vi "4155C VAR2 StartStopStep to num steps.vi"(3 "step":dbl=0.01 format="%^.4e", 4 "stop":dbl=1.0 format="%^.4e", 5 "start":dbl format="%^.4e") -> (0 "Corrected Step":dbl format="%.2f", 1 "Number of points":i32=1, 2 "dup start":dbl format="%^.4e")   [LabVIEW 2019]
doc: "Inputs the start, stop and step parameters and outputs the start, step and number of points as required for VAR2 Another wonderful display of Agilent logic.\n\nThis VI will set calculate the (integer) number of points by int((start-stop)/step)+1 and then recalculates the STEP value so the run always stops at STOP. Eg, if you have: start 0, stop 9, step 5, the program will return start 0, num steps 3, step 4.5"
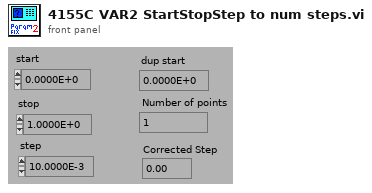
[diagram p1: front panel]
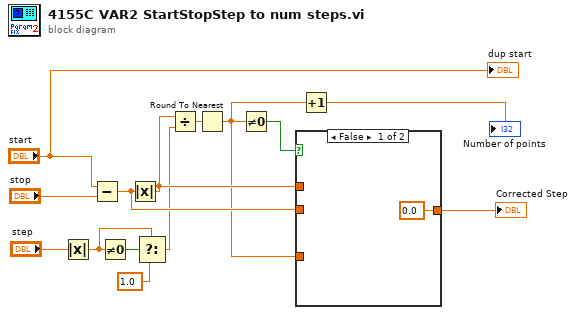
[diagram p0: block diagram]
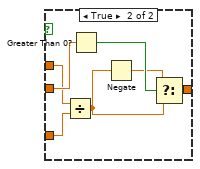
[diagram p2: hidden frame]
diagram:
  n1 = Absolute Value(x="step") -> (abs(x)=w2:dbl)
  n2 = Subtract(x="start", y="stop") -> (x-y=w13:dbl)
  n3 = Not Equal To 0?(x=w2) -> (x != 0?=w4:bool)
  n4 = Absolute Value(x=w13) -> (abs(x)=w8:dbl)
  n5 = Select(t=w2, s=w4, f=1.0) -> (s? t:f=w3:dbl)
  n6 = Divide(x=w8, y=w3) -> (x/y=w9:dbl)
  n7 = Round To Nearest(number=w9) -> (nearest integer value=w5:dbl)
  n8 = Not Equal To 0?(x=w5) -> (x != 0?=w6:bool)
  n9 = case shown="False" w6 {
    tunnel: w13 -> [_ w22]
    tunnel: [0.0 w19] -> w12
    tunnel: w8 -> [_ w18]
    tunnel: w5 -> [_ w16]
    frame False {
    }
    frame True {
      n10 = Divide(x=w18, y=w16) -> (x/y=w17:dbl)
      n11 = Greater Than 0?(x=w22) -> (x > 0?=w21:bool)
      n12 = Negate(x=w17) -> (-x=w20:dbl)
      n13 = Select(t=w20, s=w21, f=w17) -> (s? t:f=w19:dbl)
    }
  }
  "Corrected Step" <- w12
  n14 = Increment(x=w5) -> (x+1=→"Number of points":dbl)
  "dup start" <- "start"
